vi "ROI thickener.vi"(2 "error in":errorcluster, 3 "ROI Descriptor in":T2) -> (0 "error out":errorcluster, 1 "ROI Descriptor out":T1 {"Contours"."Type" items=["No Selection", "Point", "Line", "Rectangle", "Oval", "Polygon", "Freehand Region", "Annulus", "Unused2", "Unused3", "Broken Line", "Freehand Line", "Rotated Rectangle"]})   [LabVIEW 2011]
uses:
  <vilib>/vision/NI_Vision_Development_Module.lvlib
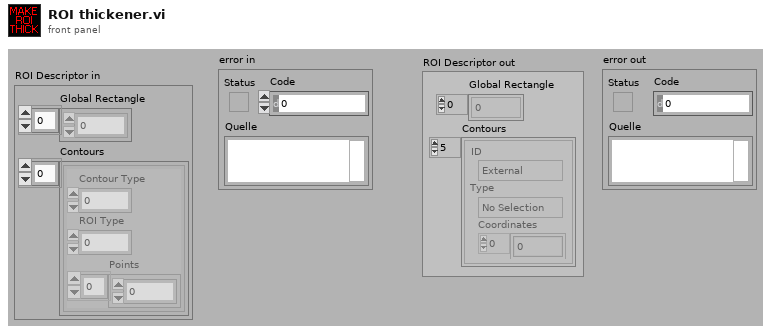
[diagram p1: front panel]
types:
  T1 = typedef "ROI Descriptor" = cluster{"Global Rectangle":i32[], "Contours":cluster{"ID":enum32{"External", "Internal"}, "Type":u32, "Coordinates":i32[]}[]}
  T2 = cluster{"Global Rectangle":i32[], "Contours":cluster{"Contour Type":u32, "ROI Type":u32, "Points":i32[]}[]}
  T3 = cluster{"Origin":cluster{"X":sgl, "Y":sgl}, "Angle (deg)":sgl, "Axis Reference":u32}
  T4 = cluster{"Global Rectangle":i32[], "Contours":cluster{"Contour Type":u32, "ROI Type":u32, "Points":i32[]}[]}[]
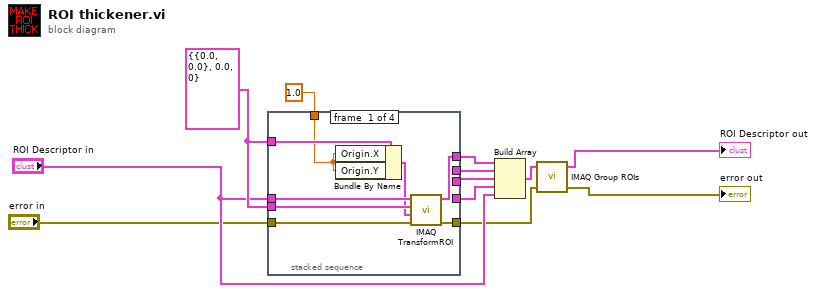
[diagram p0: block diagram]
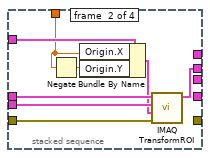
[diagram p2: hidden frame]
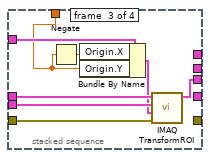
[diagram p3: hidden frame]
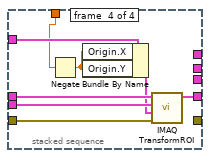
[diagram p4: hidden frame]
diagram:
  w12 = T3 {"Origin"={"X"=0.0, "Y"=0.0}, "Angle (deg)"=0.0, "Axis Reference"=0} ("Base Reference")
  n1 = stacked-sequence {
    tunnel: "error in" -> [w20 w28 w36 w44]
    tunnel: w12 -> [w19 w26 w35 w43]
    tunnel: "ROI Descriptor in" -> [w18 w25 w34 w42]
    tunnel: [w17 _ _ _] -> w2
    tunnel: [_ w24 _ _] -> w3
    tunnel: [_ _ w32 _] -> w4
    tunnel: [_ _ _ w40] -> w5
    tunnel: [w16 _ _ _] -> w9
    tunnel: w12 -> [w15 w23 w31 w39]
    tunnel: sgl 1.0 ("Origin.X") -> [w13 w21 w29 w37]
    frame #0 {
      n2 = Bundle By Name(cluster=w15, "Origin.X"=w13, "Origin.Y"=w13) -> (w14:T3)
      n3 = call "IMAQ TransformROI"("error in (no error)"=w20, "New Reference"=w14, "Base Reference"=w19, "ROI Descriptor"=w18) -> ("error out"=w16:errorcluster, "ROI Descriptor out"=w17:T1)  [unwired: 6 in]
    }
    frame #1 {
      n4 = Negate(x=w21) -> (-x=w27:sgl)
      n5 = Bundle By Name(cluster=w23, "Origin.X"=w21, "Origin.Y"=w27) -> (w22:T3)
      n6 = call "IMAQ TransformROI"("error in (no error)"=w28, "New Reference"=w22, "Base Reference"=w26, "ROI Descriptor"=w25) -> ("ROI Descriptor out"=w24:T1)  [unwired: 6 in, 1 out]
    }
    frame #2 {
      n7 = Negate(x=w29) -> (-x=w33:sgl)
      n8 = Bundle By Name(cluster=w31, "Origin.X"=w33, "Origin.Y"=w29) -> (w30:T3)
      n9 = call "IMAQ TransformROI"("error in (no error)"=w36, "New Reference"=w30, "Base Reference"=w35, "ROI Descriptor"=w34) -> ("ROI Descriptor out"=w32:T1)  [unwired: 6 in, 1 out]
    }
    frame #3 {
      n10 = Negate(x=w37) -> (-x=w41:sgl)
      n11 = Bundle By Name(cluster=w39, "Origin.X"=w41, "Origin.Y"=w41) -> (w38:T3)
      n12 = call "IMAQ TransformROI"("error in (no error)"=w44, "New Reference"=w38, "Base Reference"=w43, "ROI Descriptor"=w42) -> ("ROI Descriptor out"=w40:T1)  [unwired: 6 in, 1 out]
    }
  }
  n13 = Build Array(w2, w3, w4, w5, "ROI Descriptor in") -> (w7:T4)
  n14 = call "IMAQ Group ROIs"("error in (no error)"=w9, "ROI Descriptors"=w7) -> ("error out"=→"error out":errorcluster, "ROI Descriptor out"=→"ROI Descriptor out":T1)  [unwired: 2 in]
